vi "Time_string.vi"(0 "Input String":string) -> (1 "Error String":string, 2 "24 Hour decimal":dbl format="%.2f")   [LabVIEW 2010]
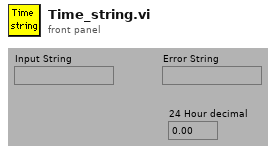
[diagram p1: front panel]
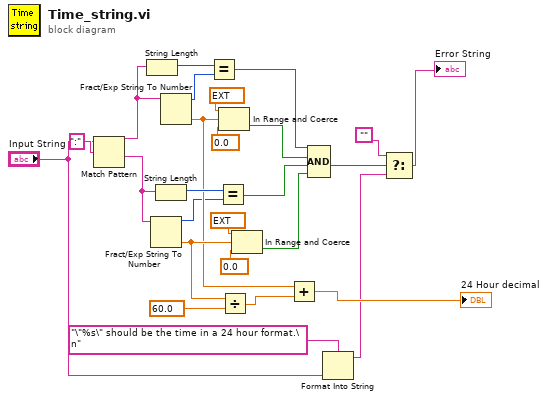
[diagram p0: block diagram]
diagram:
  n1 = Match Pattern(string="Input String", regular expression=":") -> (before substring=w12:string, after substring=w7:string)  [unwired: 3 out]
  n2 = String Length(string=w12) -> (length=w11:i32)
  n3 = Fract/Exp String To Number(string=w7) -> (offset past number=w5:i32, number=w23:dbl)  [unwired: 3 out]
  n4 = String Length(string=w7) -> (length=w8:i32)
  n5 = Fract/Exp String To Number(string=w12) -> (offset past number=w10:i32, number=w6:dbl)  [unwired: 3 out]
  n6 = Equal?(x=w11, y=w10) -> (x = y?=w9:bool)
  n7 = Equal?(x=w8, y=w5) -> (x = y?=w4:bool)
  n8 = In Range and Coerce(upper limit=ext 23.5 ("hi"), x=w6, lower limit=0.0 ("x")) -> (In Range?=w20:bool)  [unwired: 1 out]
  n9 = Divide(x=w23, y=60.0) -> (x/y=w25:dbl)
  n10 = In Range and Coerce(upper limit=ext 60.0 ("hi"), x=w23, lower limit=0.0 ("x")) -> (In Range?=w21:bool)  [unwired: 1 out]
  n11 = Add(x=w6, y=w25) -> (x+y=→"24 Hour decimal":dbl)
  n12 = Compound Arithmetic op=AND(w9, w20, w4, w21) -> (w22:bool)
  n13 = Format Into String(format string="\"%s\" should be the time in a 24 hour format.\n" ("Format String"), "Input String") -> (resulting string=w1:string)  [unwired: 2 in, 1 out]
  n14 = Select(t="", s=w22, f=w1) -> (s? t:f=→"Error String":string)
